vi "Sort Tag Combos.vi"(1 "Tag 2":T1, 2 "Tag 1":T1) -> (0 "x > y?":bool)   [LabVIEW 2025]
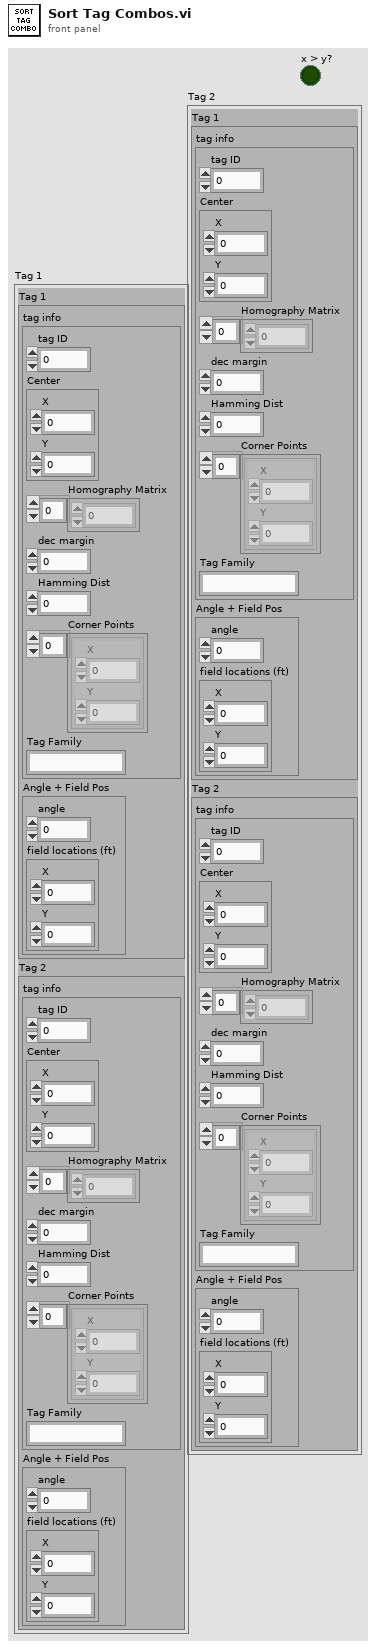
[diagram p1: front panel]
types:
  T1 = cluster{"Tag 1":cluster{"tag info":cluster{"tag ID":i32, "Center":cluster{"X":dbl, "Y":dbl}, "Homography Matrix":dbl[], "dec margin":dbl, "Hamming Dist":i32, "Corner Points":cluster{"X":dbl, "Y":dbl}[], "Tag Family":string}, "Angle + Field Pos":cluster{"angle":dbl, "field locations (ft)":cluster{"X":dbl, "Y":dbl}}}, "Tag 2":cluster{"tag info":cluster{"tag ID":i32, "Center":cluster{"X":dbl, "Y":dbl}, "Homography Matrix":dbl[], "dec margin":dbl, "Hamming Dist":i32, "Corner Points":cluster{"X":dbl, "Y":dbl}[], "Tag Family":string}, "Angle + Field Pos":cluster{"angle":dbl, "field locations (ft)":cluster{"X":dbl, "Y":dbl}}}}
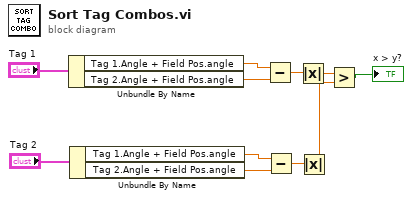
[diagram p0: block diagram]
diagram:
  n1 = Unbundle By Name("Tag 1") -> ("Tag 1.Angle + Field Pos.angle"=w10:dbl, "Tag 2.Angle + Field Pos.angle"=w11:dbl)
  n2 = Unbundle By Name("Tag 2") -> ("Tag 1.Angle + Field Pos.angle"=w3:dbl, "Tag 2.Angle + Field Pos.angle"=w2:dbl)
  n3 = Subtract(x=w10, y=w11) -> (x-y=w9:dbl)
  n4 = Subtract(x=w3, y=w2) -> (x-y=w4:dbl)
  n5 = Absolute Value(x=w9) -> (abs(x)=w8:dbl)
  n6 = Absolute Value(x=w4) -> (abs(x)=w1:dbl)
  n7 = Greater?(x=w8, y=w1) -> (0:→"x > y?":bool)
